vi "探头窗口-2.vi"() -> ()   [LabVIEW 2017]
panel:
  in  "更新数据":T1
  in  "停止信号":bool=TRUE
  out "引用-切回列表模式？":refnum<vi>
  out "更新数据？":bool=TRUE
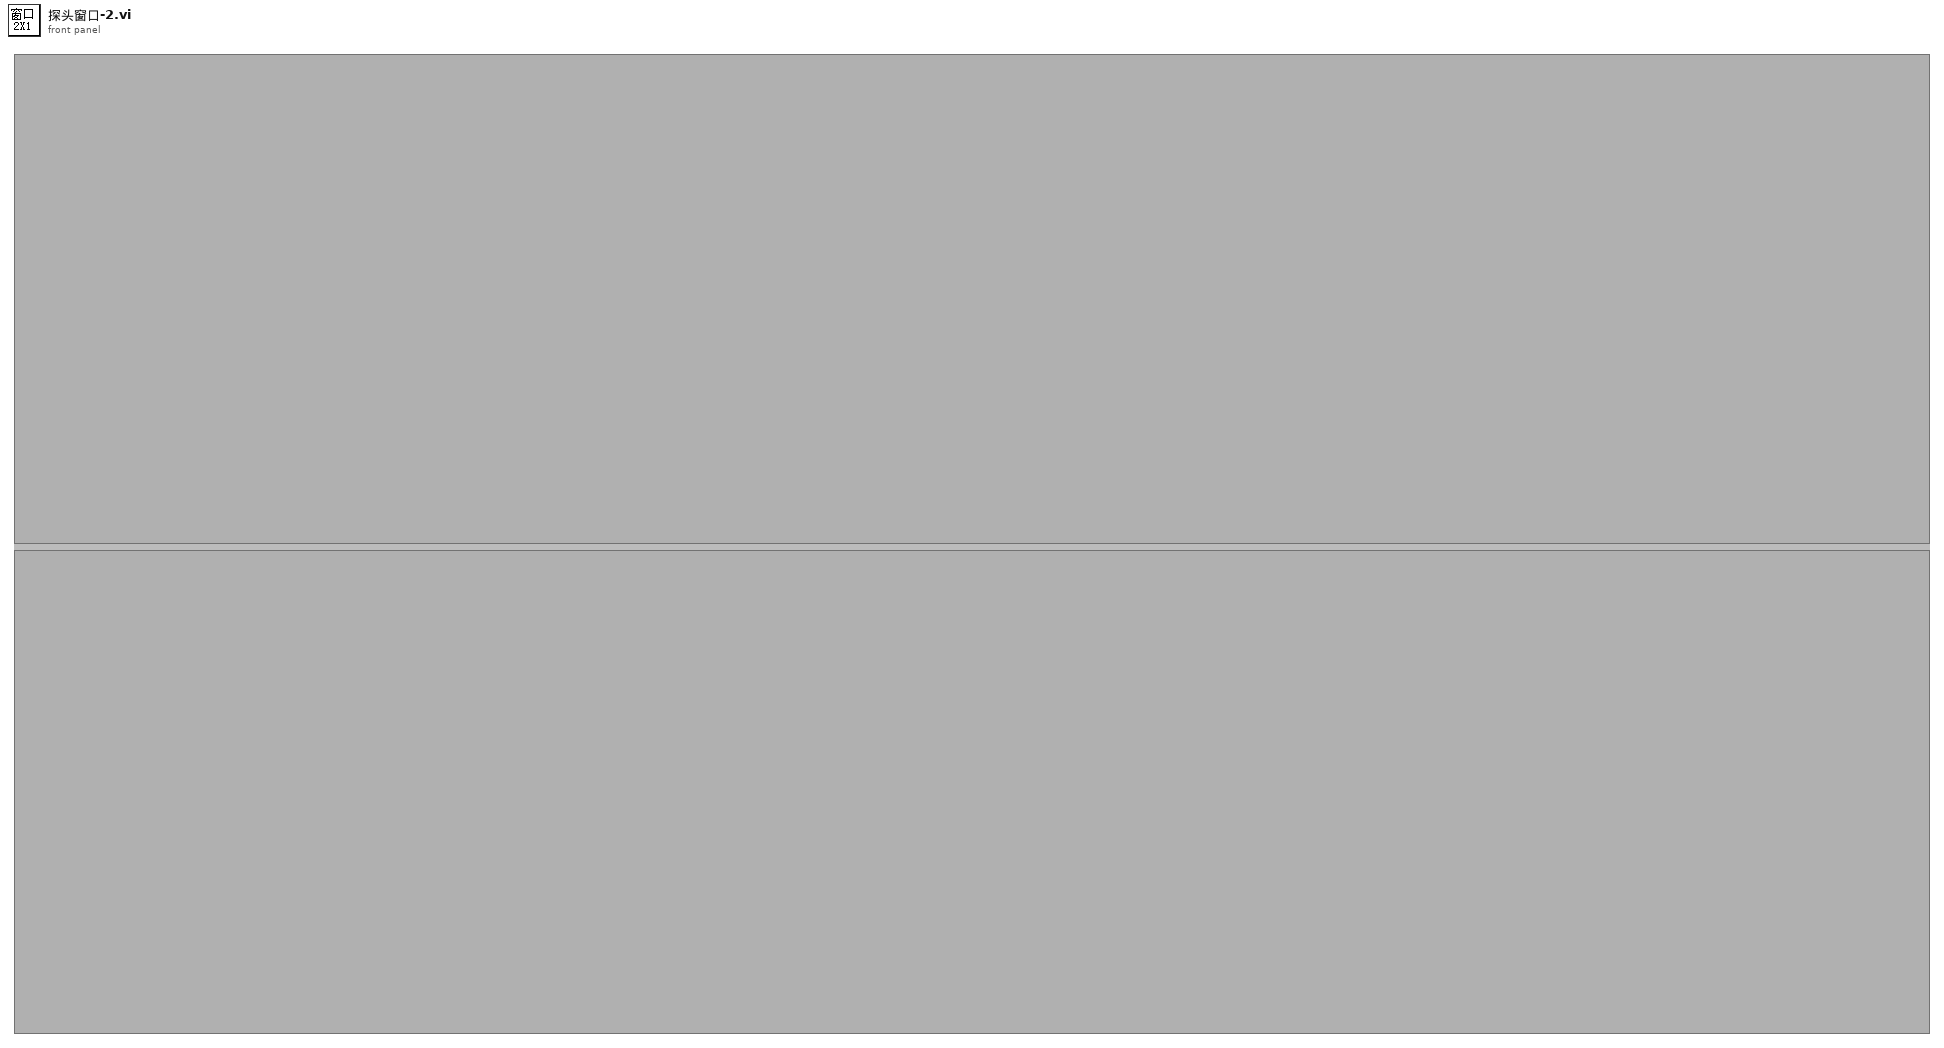
[diagram p1: front panel]
types:
  T1 = cluster{"探头启用状态？":bool[], "测量值":cluster{"X":timestamp, "Y":dbl}[], "限值":cluster{"限值1":dbl, "限值2":dbl, "探头限值":enum16{"一级限值", "二级限值"}}[], "报警状态":enum16{"正常", "一级报警", "二级报警", "累积报警"}[], "探头信息":string[], "累积剂量":cluster{"设备名称":string, "启用累积？":bool, "起始时间":timestamp, "累积剂量":dbl, "累积报警阈值":dbl}[]}
  T2 = enum32{"Invalid", "Standard", "Closed", "Hidden", "Minimized", "Maximized"}
  T3 = cluster{"启用状态？":bool, "测量值":cluster{"X":timestamp, "Y":dbl}, "限值簇":cluster{"限值1":dbl, "限值2":dbl, "探头限值":enum16{"一级限值", "二级限值"}}, "报警状态":enum16{"正常", "一级报警", "二级报警", "累积报警"}, "探头信息":string, "探头地址":i32, "累积剂量":cluster{"设备名称":string, "启用累积？":bool, "起始时间":timestamp, "累积剂量":dbl, "累积报警阈值":dbl}}
  T4 = typedef "eventvkey.ctl" = enum16{"ASCII", "Enter", "Return", "Shift", "Ctrl", "Alt", "Cmd", "Opt", "Caps", "NumLock", "Clear", "Break", "Up", "Down", "Left", "Right", "Insert", "Delete", "Home", "End", "PageUp", "PageDown", "Escape", "Help", "Pause", "ScrollLock", "F1", "F2", "F3", "F4", "F5", "F6", "F7", "F8", "F9", "F10", "F11", "F12", "F13", "F14", "F15", "F16", "F17", "F18", "F19", "F20", "F21", "F22", "F23", "F24", "Play", "VolumeUp", "VolumeDown", "Mute", "Two Byte Char"}
  T5 = cluster{"限值1":dbl, "限值2":dbl, "探头限值":enum16{"一级限值", "二级限值"}}
  T6 = cluster{"限值1":dbl, "限值2":dbl, "探头限值":enum16{"一级限值", "二级限值"}}[]
  T7 = cluster{"设备名称":string, "启用累积？":bool, "起始时间":timestamp, "累积剂量":dbl, "累积报警阈值":dbl}[]
  T8 = cluster{"设备名称":string, "启用累积？":bool, "起始时间":timestamp, "累积剂量":dbl, "累积报警阈值":dbl}
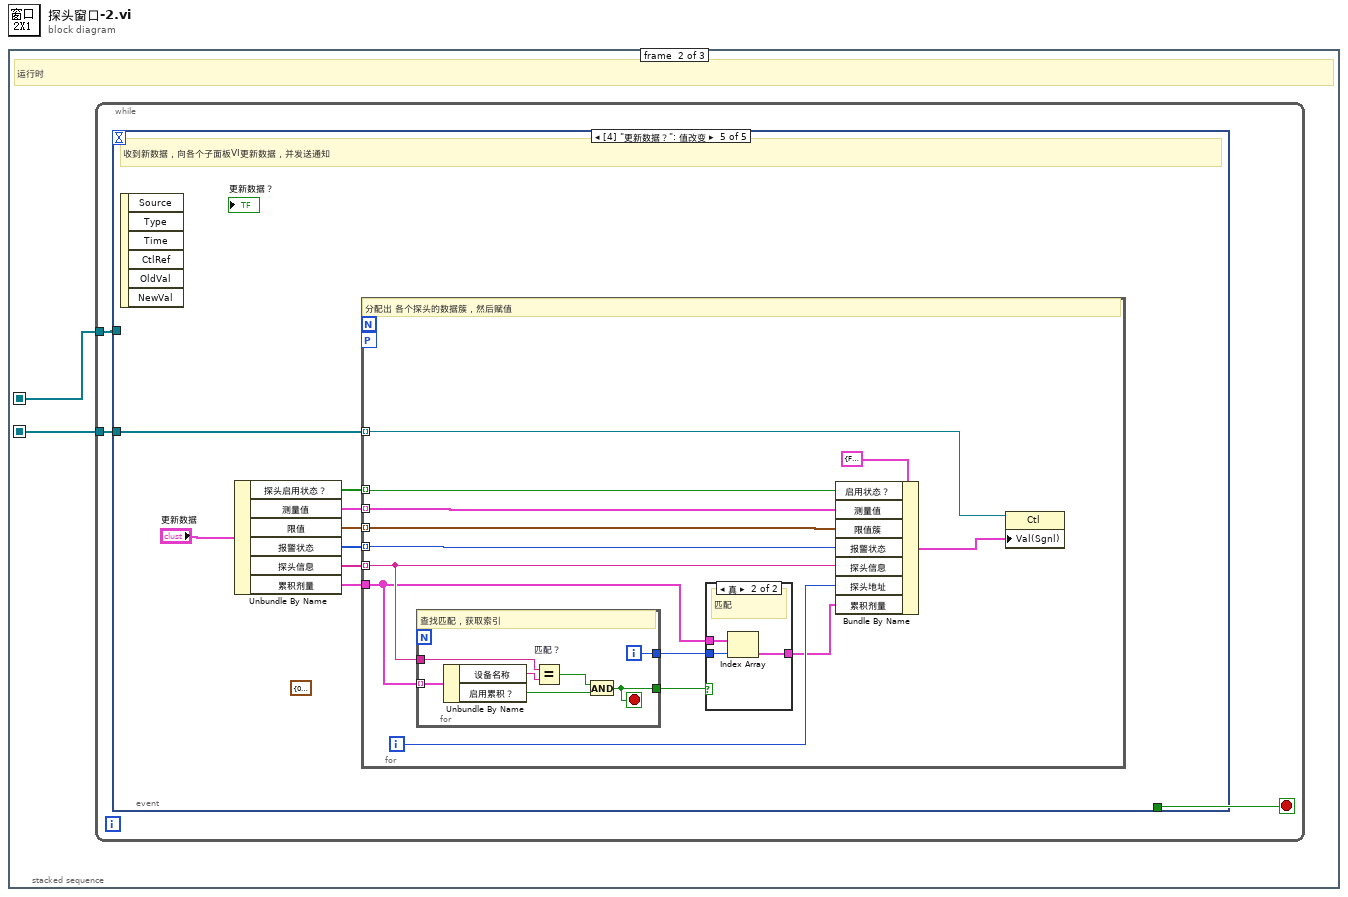
[diagram p0: block diagram]
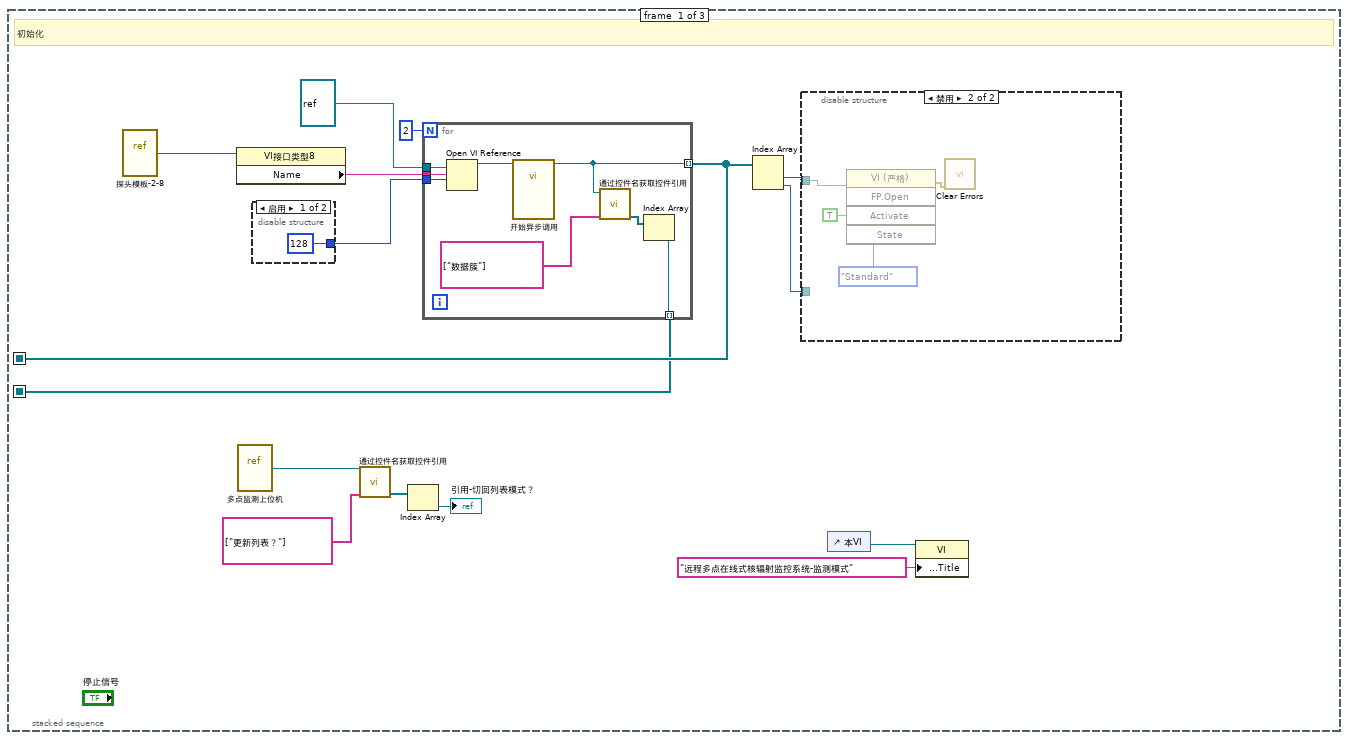
[diagram p2: hidden frame]
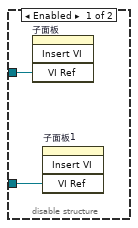
[diagram p3: hidden frame]
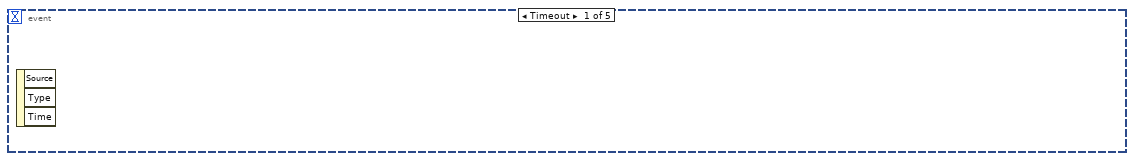
[diagram p5: hidden frame]
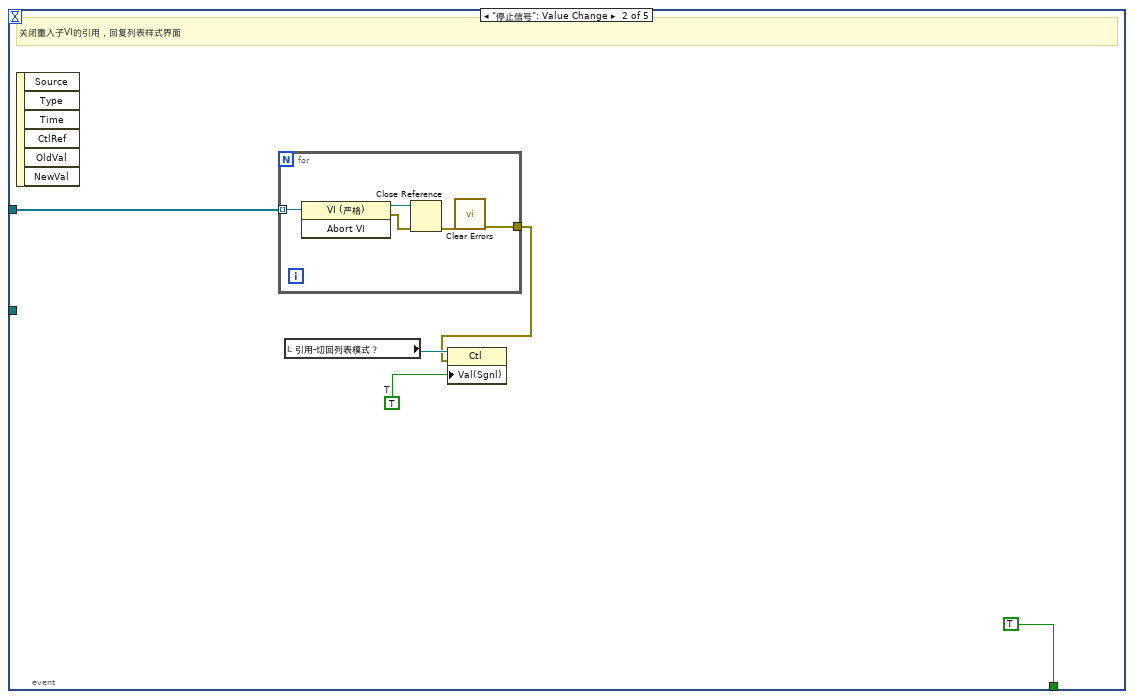
[diagram p6: hidden frame]
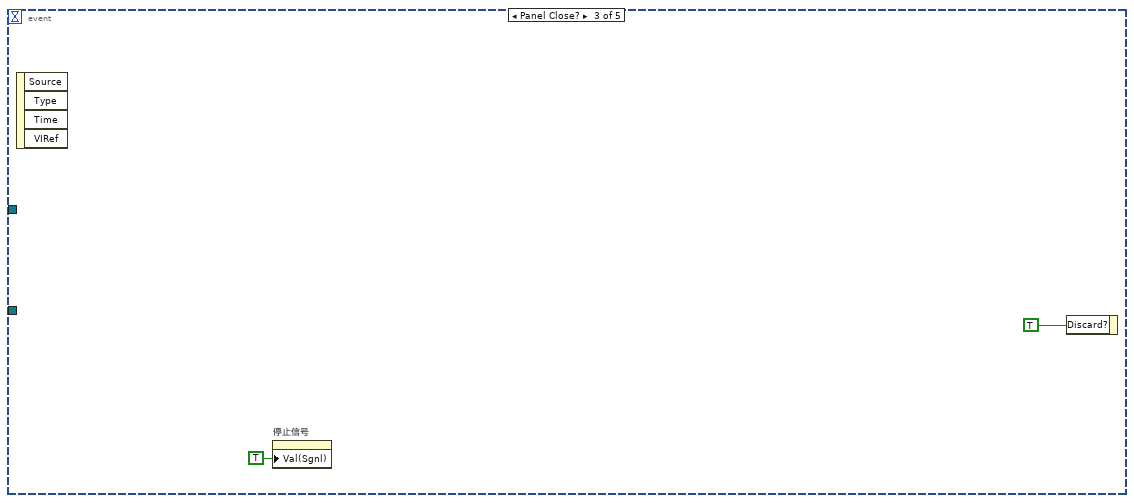
[diagram p7: hidden frame]
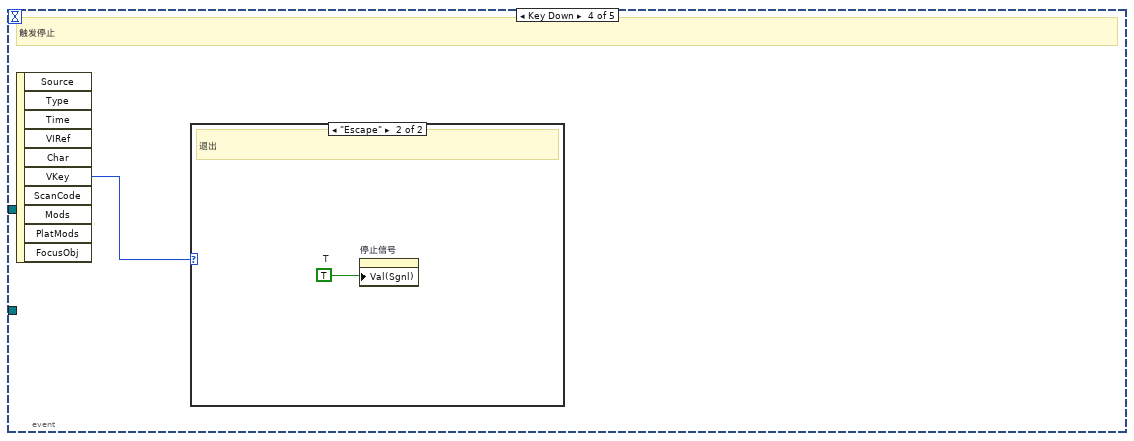
[diagram p8: hidden frame]
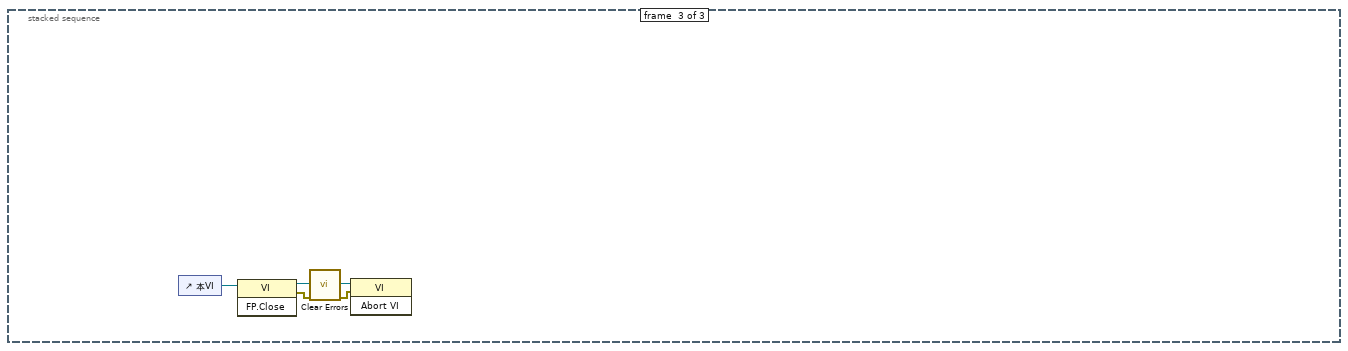
[diagram p11: hidden frame]
diagram:
  n1 = stacked-sequence {
    seq-local: [w11 _ _] -> [_ w32 _]
    seq-local: [w3 _ _] -> [_ w31 _]
    frame #0 {
      # "初始化"
      n2 = vi-ref "探头模板-2-8.vi"() -> (w15:refnum<vi>)
      n3 = property class="VI接口类型8"(reference=w15) -> ("Name"=w14:string)  [unwired: 1 in, 2 out]
      n4 = vi-ref "多点监测上位机.vi"() -> (w7:refnum<vi>)
      n5 = disable-structure shown="启用" {
        disable-tunnel: [128 ("选项") _] -> w13
        frame Enabled {
        }
        frame Disabled {
        }
      }
      n6 = call "通过控件名获取控件引用.vi"("控件名数组"=string[] ["更新列表？"], "VI引用"=w7) -> ("控件引用输出"=w5:refnum<vi>[])  [unwired: 7 in, 2 out]
      n7 = Index Array(array=w5) -> (element=→"引用-切回列表模式？":refnum<vi>)  [unwired: 1 in]
      n8 = for {
        N: 2 -> [_]
        tunnel: w14 -> [w30]
        tunnel: w13 -> [w29]
        tunnel: refnum<vi> refnum ("类型说明符VI引用句柄（仅用于类型）") -> [w28]
        tunnel: [w23] -> w11 mode=indexing
        tunnel: [w24] -> w3 mode=indexing
        n9 = Open VI Reference(type specifier VI Refnum (for type only)=w28, vi path=w30, options=w29) -> (vi reference=w27:refnum<vi>)  [unwired: 3 in, 1 out]
        n10 = call-by-ref "开始异步调用"(reference=w27) -> (reference out=w23:refnum<vi>)  [unwired: 13 in, 1 out]
        n11 = call "通过控件名获取控件引用.vi"("控件名数组"=string[] ["数据簇"], "VI引用"=w23) -> ("控件引用输出"=w25:refnum<vi>[])  [unwired: 7 in, 2 out]
        n12 = Index Array(array=w25) -> (element=w24:refnum<vi>)  [unwired: 1 in]
      }
      n13 = Index Array(array=w11) -> (element #1=w10:refnum<vi>, element #2=w9:refnum<vi>)  [unwired: 2 in]
      n14 = disable-structure shown="禁用" {
        disable-tunnel: w10 -> [w16 w21]
        disable-tunnel: w9 -> [w17 _]
        frame Enabled {
          n15 = invoke on="子面板" class="子面板" method="Insert VI"("VI Ref"=w16) -> ()  [unwired: 3 in, 4 out]
          n16 = invoke on="子面板1" class="SubPnl" method="Insert VI"("VI Ref"=w17) -> ()  [unwired: 3 in, 4 out]
        }
        frame Disabled {
          n17 = invoke class="VI (严格)" method="FP.Open"(reference=w21, "Activate"=TRUE ("激活？"), "State"=T2."Standard" ("状态")) -> (error out=w18:errorcluster)  [unwired: 2 in, 4 out]
          n18 = call <vilib>:"Clear Errors.vi"("error in (no error)"=w18) -> ()  [unwired: 5 in, 2 out]
        }
      }
      n19 = control-ref of="本VI"() -> (w2:refnum<vi>)
      n20 = property class="VI"(reference=w2, "Front Panel.Title"="远程多点在线式核辐射监控系统-监测模式" ("前面板窗口:标题")) -> ()  [unwired: 1 in, 2 out]
    }
    frame #1 {
      # "运行时"
      n21 = while {
        tunnel: w32 -> [w34]
        tunnel: w31 -> [w33]
        stop <- w35 stop-if-true
        n22 = event shown="[4] \"更新数据？\": 值改变" {
          selector: _ -> [_ _ _ _ _]
          dyn-events: _ -> [_ _ _ _ _]
          timeout: _ -> [_ _ _ _ _]
          tunnel: [_ TRUE ("放弃？") _ _ _] -> w35
          tunnel: w34 -> [_ w40 _ _ _]
          tunnel: w33 -> [_ _ _ _ w52]
          event Timeout {
            n23 = event-data() -> ()  [unwired: 1 in, 3 out]
          }
          event "停止信号": Value Change {
            w38 = TRUE  # T
            # "关闭重入子VI的引用，回复列表样式界面"
            n24 = event-data() -> ()  [unwired: 1 in, 6 out]
            n25 = for {
              tunnel: w40 -> [w45] mode=indexing
              tunnel: [w41] -> w37
              n26 = invoke class="VI (严格)" method="Abort VI"(reference=w45) -> (reference out=w43:refnum<vi>, error out=w44:errorcluster)  [unwired: 2 in, 1 out]
              n27 = Close Reference(reference=w43, error in (no error)=w44) -> (error out=w42:errorcluster)
              n28 = call <vilib>:"Clear Errors.vi"("error in (no error)"=w42) -> ("error out"=w41:errorcluster)  [unwired: 5 in, 1 out]
            }
            n29 = local read "引用-切回列表模式？"() -> (w39:refnum<vi>)
            n30 = property class="Ctl"(reference=w39, error in=w37, "Val(Sgnl)"=w38) -> ()  [unwired: 2 out]
          }
          event Panel Close? {
            n31 = event-data() -> ()  [unwired: 1 in, 4 out]
            n32 = property on="停止信号" class="Bool (严格)"("Val(Sgnl)"=TRUE ("值(信号)")) -> ()  [unwired: 2 in, 2 out]
            n33 = event-data("Discard?"=TRUE ("放弃？")) -> ()  [unwired: 1 in, 1 out]
          }
          event Key Down {
            # "触发停止"
            n34 = event-data() -> ("VKey"=w48:T4)  [unwired: 1 in, 9 out]
            n35 = case shown="\"Escape\"" w48 {
              frame "ASCII", Default {
              }
              frame "Escape" {
                w49 = TRUE  # T
                # "退出"
                n36 = property on="停止信号" class="Bool (严格)"("Val(Sgnl)"=w49) -> ()  [unwired: 2 in, 2 out]
              }
            }
          }
          event "更新数据？": Value Change {
            (unwired) T5 {"限值1"=0.0, "限值2"=0.0, "探头限值"=enum."一级限值"} ("探头限值簇")
            # "收到新数据，向各个子面板VI更新数据，并发送通知"
            n37 = event-data() -> ()  [unwired: 1 in, 6 out]
            n38 = Unbundle By Name("更新数据") -> ("探头启用状态？"=w57:bool[], "测量值"=w56:cluster{"X":timestamp, "Y":dbl}[], "限值"=w55:T6, "报警状态"=w54:enum16{"正常", "一级报警", "二级报警", "累积报警"}[], "探头信息"=w53:string[], "累积剂量"=w51:T7)
            n39 = for {
              tunnel: w57 -> [w70] mode=indexing
              tunnel: w56 -> [w69] mode=indexing
              tunnel: w55 -> [w68] mode=indexing
              tunnel: w54 -> [w67] mode=indexing
              tunnel: w53 -> [w62] mode=indexing
              workers-P: _ -> [_]
              tunnel: w52 -> [w65] mode=indexing
              tunnel: w51 -> [w61]
              i -> [w63]
              # "分配出 各个探头的数据簇，然后赋值"
              n40 = for {
                tunnel: w61 -> [w80] mode=indexing
                tunnel: w62 -> [w78]
                tunnel: [w75] -> w60
                tunnel: [w74] -> w59
                i -> [w75]
                stop <- w74 stop-if-true
                # "查找匹配，获取索引"
                n41 = Unbundle By Name(w80) -> ("设备名称"=w79:string, "启用累积？"=w76:bool)
                n42 = Equal? "匹配？"(x=w78, y=w79) -> (x = y?=w77:bool)
                n43 = And(x=w77, y=w76) -> (x .and. y?=w74:bool)
              }
              n44 = case shown="真" w59 {
                tunnel: w61 -> [_ w73]
                tunnel: w60 -> [_ w72]
                tunnel: [_ w71] -> w58
                frame False {
                  # "不匹配"
                }
                frame True {
                  # "匹配"
                  n45 = Index Array(array=w73, index=w72) -> (element=w71:T8)
                }
              }
              n46 = Bundle By Name(cluster=T3 {"启用状态？"=FALSE, "测量值"={"X"=timestamp(0 s since 1904-01-01), "Y"=0.0}, "限值簇"={"限值1"=0.0, "限值2"=0.0, "探头限值"=enum."一级限值"}, "报警状态"=enum."正常", "探头信息"="", "探头地址"=0, "累积剂量"={"设备名称"="", "启用累积？"=FALSE, "起始时间"=timestamp(0 s since 1904-01-01), "累积剂量"=0.0, "累积报警阈值"=0.0}} ("输出簇"), "启用状态？"=w70, "测量值"=w69, "限值簇"=w68, "报警状态"=w67, "探头信息"=w62, "探头地址"=w63, "累积剂量"=w58) -> (w64:T3)
              n47 = property class="Ctl"(reference=w65, "Val(Sgnl)"=w64) -> ()  [unwired: 1 in, 2 out]
            }
          }
        }
      }
    }
    frame #2 {
      n48 = control-ref of="本VI"() -> (w84:refnum<vi>)
      n49 = invoke class="VI" method="FP.Close"(reference=w84) -> (reference out=w83:refnum<vi>, error out=w81:errorcluster)  [unwired: 2 in, 1 out]
      n50 = call <vilib>:"Clear Errors.vi"("error in (no error)"=w81) -> ("error out"=w82:errorcluster)  [unwired: 5 in, 1 out]
      n51 = invoke class="VI" method="Abort VI"(reference=w83, error in=w82) -> ()  [unwired: 1 in, 3 out]
    }
  }
